vi "set_pixel_dwell_time.vi"(8 "error in (no error)":errorcluster, 10 "pixel dwell time":dbl[unit], 11 "FPGAWrapperMH120124FrameScan_PXI7813R in":refnum<class "FPGAWrapperMH120124FrameScan_PXI7813R.lvclass">) -> (0 "error out":errorcluster, 3 "FPGAWrapperMH120124FrameScan_PXI7813R out":refnum<class "FPGAWrapperMH120124FrameScan_PXI7813R.lvclass">)   [LabVIEW 2010, in "FPGAWrapperMH120124FrameScan_PXI7813R.lvclass"]
uses:
  FPGAWrapperMH120124FrameScan_PXI7813R.lvclass
  FPGAWrapperMH120124FrameScan_PXI7813R.lvclass/FPGAWrapperMH120124FrameScan_PXI7813R.ctl
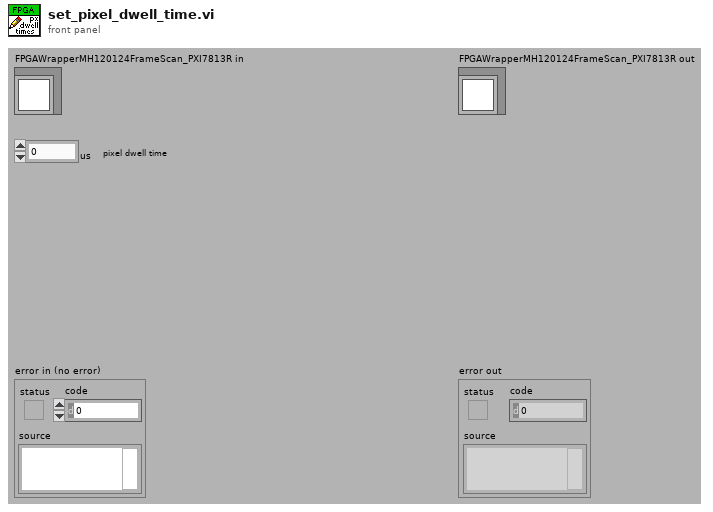
[diagram p1: front panel]
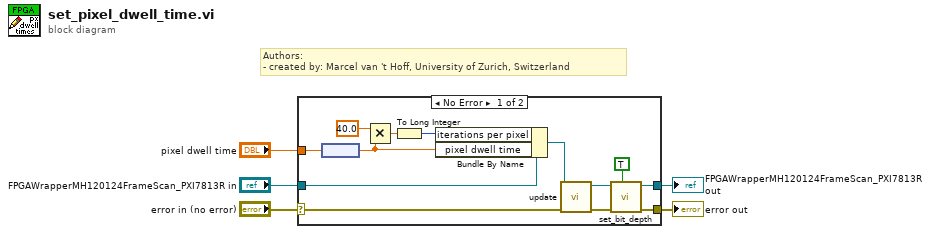
[diagram p0: block diagram]
diagram:
  # "Authors: \n- created by: Marcel van 't Hoff, University of Zurich, Switzerland"
  n1 = case shown="No Error" "error in (no error)" {
    selector: "error in (no error)" -> [w12 w19]
    tunnel: [w7 w19] -> w4
    tunnel: [w9 w20] -> w2
    tunnel: "FPGAWrapperMH120124FrameScan_PXI7813R in" -> [w18 w20]
    tunnel: "pixel dwell time" -> [w17 _]
    frame No Error {
      n2 = node(w17) -> (w16:dbl)
      n3 = Multiply(x=40.0, y=w16) -> (x*y=w14:dbl)
      n4 = To Long Integer(number=w14) -> (32bit integer=w13:i32)
      n5 = Bundle By Name(cluster=w18, "iterations per pixel"=w13, "pixel dwell time"=w16) -> (w11:refnum<class "FPGAWrapperMH120124FrameScan_PXI7813R.lvclass">)
      n6 = call-dynamic "update.vi"("error in (no error)"=w12, "FPGAWrapperMH120124FrameScan_PXI7813R in"=w11) -> ("error out"=w8:errorcluster, "FPGAWrapperMH120124FrameScan_PXI7813R out"=w10:refnum<class "FPGAWrapperMH120124FrameScan_PXI7813R.lvclass">)  [unwired: 8 in]
      n7 = call-dynamic "set_bit_depth.vi"("calculate by timing? (F)"=TRUE, "error in (no error)"=w8, "FPGAWrapperMH120124FrameScan_PXI7813R in"=w10) -> ("error out"=w7:errorcluster, "FPGAWrapperMH120124FrameScan_PXI7813R out"=w9:refnum<class "FPGAWrapperMH120124FrameScan_PXI7813R.lvclass">)  [unwired: 7 in]
    }
    frame Error {
    }
  }
  "error out" <- w4
  "FPGAWrapperMH120124FrameScan_PXI7813R out" <- w2
